vi "AutoDrive.vi"(9 "Steady Val":dbl, 11 "Distance to travel (inches)":dbl) -> ()   [LabVIEW 2013]
uses:
  Robot Global Data.vi
  State_Machine_Enum.ctl
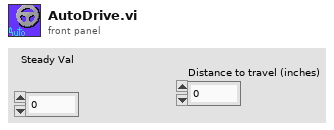
[diagram p1: front panel]
types:
  T1 = typedef "State_Machine_Enum.ctl" = enum16{"Idle", "Start", "Do", "Stop", "Init"}
  T2 = typedef "LoopDisable.ctl" = cluster{"Climb.vi":bool, "LauncherAngle.vi":bool, "Launcher.vi":bool, "ArmControl.vi":bool, "WinchMotor.vi":bool, "ReadDriveEncoder.vi":bool}
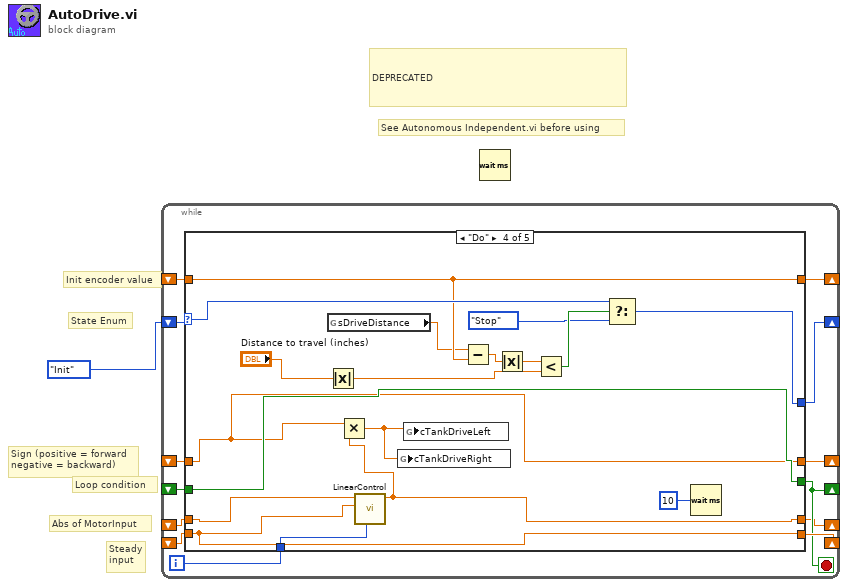
[diagram p0: block diagram]
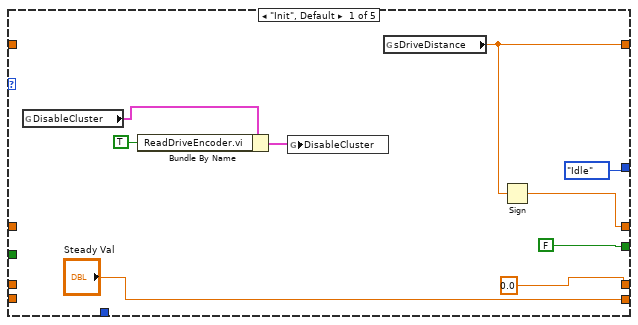
[diagram p2: hidden frame]
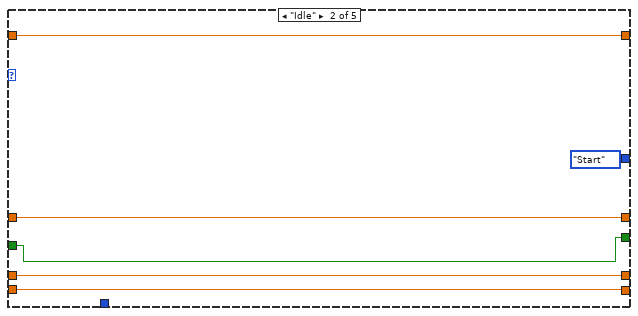
[diagram p3: hidden frame]
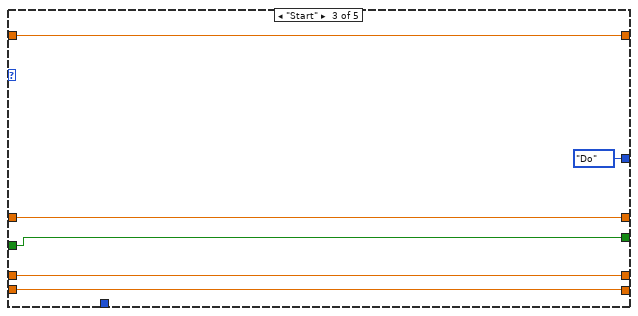
[diagram p4: hidden frame]
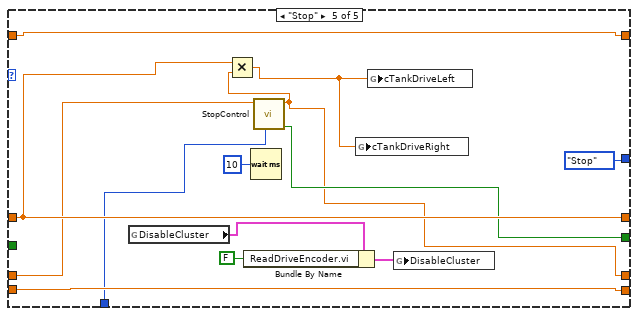
[diagram p5: hidden frame]
diagram:
  # "See Autonomous Independent.vi before using"
  # "DEPRECATED"
  # "Sign (positive = forward\nnegative = backward)"
  # "Init encoder value"
  # "State Enum"
  # "Loop condition"
  # "Abs of MotorInput"
  # "Steady\ninput"
  n1 = while {
    shift-right: [w13] -> _
    shift-left: State_Machine_Enum."Init" ("State") -> [w14]
    shift-right: [w12] -> _
    shift-left: _ -> [w11]
    shift-right: [w10] -> _
    shift-left: _ -> [w9]
    shift-right: [w8] -> _
    shift-left: _ -> [w7]
    shift-right: [w6] -> _
    shift-left: _ -> [w5]
    shift-right: [w4] -> _
    shift-left: _ -> [w3]
    i -> [w2]
    stop <- w10 stop-if-true
    n2 = case shown="\"Do\"" w14 {
      selector: w14 -> [_ _ _ w53 _]
      tunnel: [State_Machine_Enum."Idle" ("State") State_Machine_Enum."Start" ("State") State_Machine_Enum."Do" ("State") w52 State_Machine_Enum."Stop" ("State")] -> w13
      tunnel: ["Steady Val" w29 w35 w49 w66] -> w12
      tunnel: w11 -> [_ w29 w35 w49 w66]
      tunnel: [FALSE w28 w34 w47 w55] -> w10
      tunnel: w9 -> [_ w28 w34 w47 _]
      tunnel: [0.0 ("New Motor Input") w27 w33 w45 w54] -> w8
      tunnel: w7 -> [_ w27 w33 w46 w56]
      tunnel: [w17 w26 w32 w40 w65] -> w6
      tunnel: w5 -> [_ w26 w32 w40 w65]
      tunnel: [w16 w24 w30 w41 w63] -> w4
      tunnel: w3 -> [_ w24 w30 w41 w63]
      tunnel: w2 -> [_ _ _ w36 w57]
      frame "Init", Default {
        n3 = global read "Robot Global Data.vi" "DisableCluster"() -> (w20:T2)
        n4 = Bundle By Name(cluster=w20, "ReadDriveEncoder.vi"=TRUE) -> (w18:T2)
        n5 = global write "Robot Global Data.vi" "DisableCluster"(w18) -> ()
        n6 = global read "Robot Global Data.vi" "sDriveDistance"() -> (w17:dbl)
        n7 = Sign(1:w17) -> (0:w16:dbl)
      }
      frame "Idle" {
      }
      frame "Start" {
      }
      frame "Do" {
        n8 = global read "Robot Global Data.vi" "sDriveDistance"() -> (w39:dbl)
        n9 = Absolute Value(x="Distance to travel (inches)") -> (abs(x)=w42:dbl)
        n10 = call "LinearControl.vi"("Loop Iteration"=w36, "Setpoint"=w49, "Motor Value"=w46) -> ("New Motor Value"=w45:dbl)  [unwired: 7 in, 1 out]
        n11 = Multiply(x=w41, y=w45) -> (x*y=w37:dbl)
        n12 = global write "Robot Global Data.vi" "cTankDriveRight"(w37) -> ()
        n13 = global write "Robot Global Data.vi" "cTankDriveLeft"(w37) -> ()
        n14 = Subtract(x=w39, y=w40) -> (x-y=w44:dbl)
        n15 = Absolute Value(x=w44) -> (abs(x)=w38:dbl)
        n16 = Less?(x=w38, y=w42) -> (x < y?=w50:bool)
        n17 = Select(t=w53, s=w50, f=State_Machine_Enum."Stop" ("State")) -> (s? t:f=w52:T1)
        n18 = Wait (ms)(milliseconds to wait=u32 10) -> ()  [unwired: 1 out]
      }
      frame "Stop" {
        n19 = global read "Robot Global Data.vi" "DisableCluster"() -> (w62:T2)
        n20 = Bundle By Name(cluster=w62, "ReadDriveEncoder.vi"=FALSE) -> (w60:T2)
        n21 = Wait (ms)(milliseconds to wait=u32 10) -> ()  [unwired: 1 out]
        n22 = call "StopControl.vi"("Loop Iteration"=w57, "Motor Value"=w56) -> ("Done Stopping"=w55:bool, "New Motor Value"=w54:dbl)  [unwired: 8 in]
        n23 = Multiply(x=w63, y=w54) -> (x*y=w59:dbl)
        n24 = global write "Robot Global Data.vi" "cTankDriveRight"(w59) -> ()
        n25 = global write "Robot Global Data.vi" "cTankDriveLeft"(w59) -> ()
        n26 = global write "Robot Global Data.vi" "DisableCluster"(w60) -> ()
      }
    }
  }
  n27 = Wait (ms)() -> ()  [unwired: 1 in, 1 out]
